vi "Main.vi"() -> ()   [LabVIEW 2024]
doc: "Use this template to build a simple state machine design pattern. Each state executes code and determines which state to transition to."
uses:
  controls/Valves--cluster.ctl
  controls/Controls--cluster.ctl
  controls/Sensors--cluster.ctl
  controls/SystemInfo--cluster.ctl
  <vilib>/gRPC/LabVIEW gRPC Library/Shared/grpcId.ctl
  controls/UI Queue Element.ctl
  controls/States.ctl
  controls/Stream Queue Element.ctl
  controls/Stream Loop States.ctl
  pumploop_client/RPC Messages/pumploop_GetSysInfRequest.ctl
  pumploop_client/RPC Messages/pumploop_GetValveRequest.ctl
  pumploop_client/RPC Messages/pumploop_GetControlRequest.ctl
  pumploop_client/RPC Messages/pumploop_Controls.ctl
  pumploop_client/RPC Messages/pumploop_Valves.ctl
  pumploop_client/RPC Messages/pumploop_GetSensorRequest.ctl
  pumploop_client/pumploop_client.lvlib
  <vilib>/gRPC/LabVIEW gRPC Library/grpc-lvsupport-release.lvlib
  pumploop_client/RPC Messages/pumploop_SystemInfo.ctl
panel:
  out "Read Attempts":i32
  out "Successes":bool[](array[boolean])
  in  "Apply Preset":bool
  in  "Address Presets":enum16{"Home WiFi", "RasPi WiFi"}(ring)
  out "Stream Status":string
  out "Stream Response Graph":waveform(dbl)[](graph)
  in  "Stream Enable":bool
  out "Node Info":T1
  out "Sensors":T2 {"Pump Speed" scale=0.0..10.0; "Ambient Pressure" scale=0.5..1.5; "DUT Outlet Pressure" scale=0.0..5.0; "DUT Inlet Pressure" scale=0.0..10.0; "Flow" scale=0.0..100.0; "Sump Level" scale=0.0..100.0; "Tank Level" scale=0.0..100.0; "DUT Temp" scale=0.0..150.0; "Pump Temp" scale=0.0..150.0; "Tank Temp" scale=0.0..100.0; "Ambient Temp" scale=0.0..50.0}
  in  "Get/Set":enum16{"Get", "Set"}(ring)
  in  "Subsystem":T3(ring)
  in  "Stream":enum16{"Disabled", "Enabled"}(ring)
  in  "Stop":bool
  in  "gRPC Disconnect":bool
  in  "Server Address":string="10.42.0.1:50051"
  in  "gRPC Connect":bool
  in  "Pump Control":T4
  in  "Control Valves":T5
  out "gRPC ID Out":u64
  out "Error":errorcluster
  # "Open"
  # "Closed"
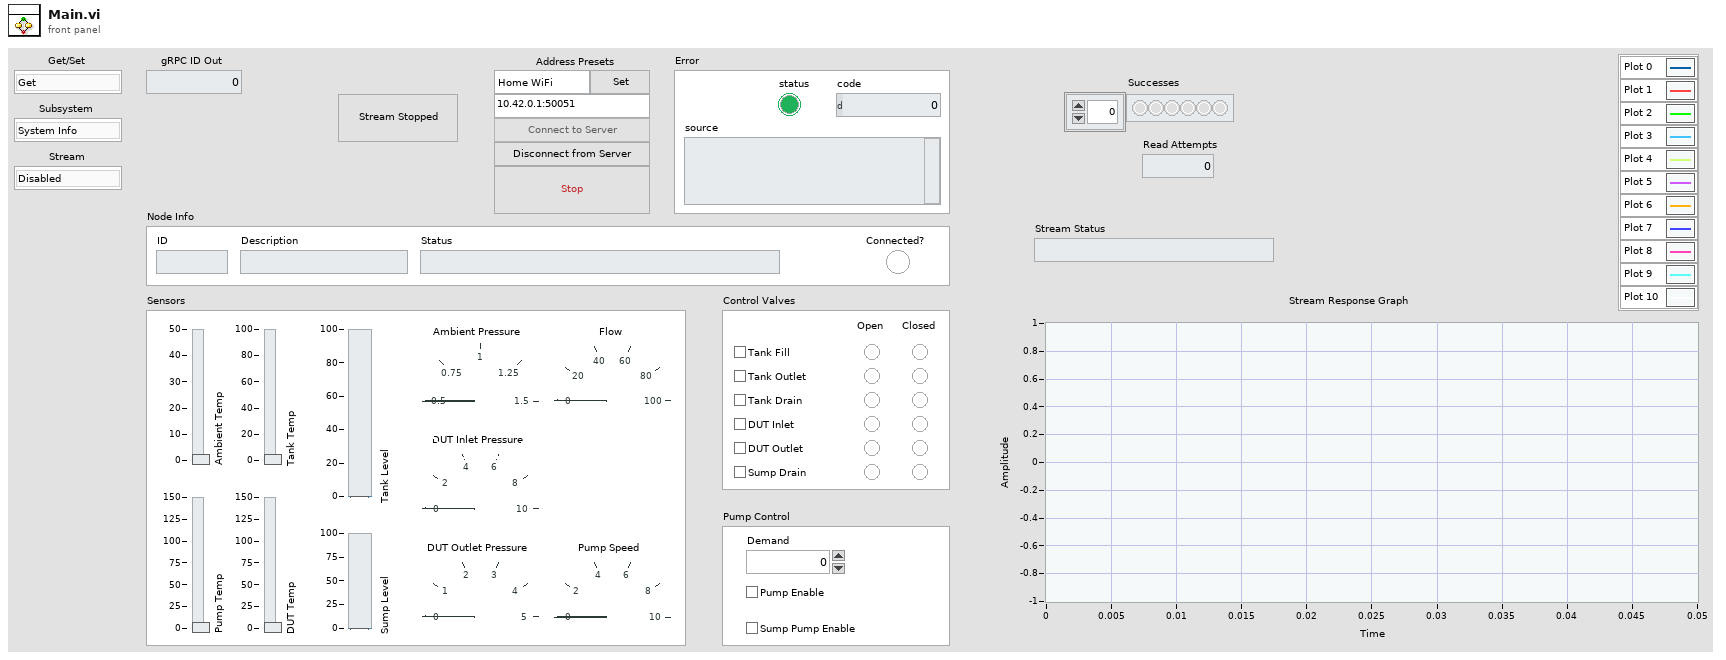
[diagram p1: front panel]
types:
  T1 = typedef "SystemInfo--cluster.ctl" = cluster{"Connected?":bool, "ID":string, "Description":string, "Status":string}
  T2 = typedef "Sensors--cluster.ctl" = cluster{"Tank Level":dbl, "Tank Temp":dbl, "Flow":dbl, "Pump Temp":dbl, "Pump Speed":dbl, "DUT Inlet Pressure":dbl, "DUT Outlet Pressure":dbl, "DUT Temp":dbl, "Sump Level":dbl, "Ambient Temp":dbl, "Ambient Pressure":dbl}
  T3 = enum16{"System Info", "Valves", "Sensors", "Control"}
  T4 = typedef "Controls--cluster.ctl" = cluster{"Pump Enable":bool, "Demand":dbl, "Sump Pump Enable":bool}
  T5 = typedef "Valves--cluster.ctl" = cluster{"Tank Fill":bool, "Tank Outlet":bool, "Tank Drain":bool, "DUT Inlet":bool, "DUT Outlet":bool, "Sump Drain":bool, "Tank Fill Open":bool, "Tank Fill Closed":bool, "Tank Outlet Open":bool, "Tank Outlet Closed":bool, "Tank Drain Open":bool, "Tank Drain Closed":bool, "DUT Inlet Open":bool, "DUT Inlet Closed":bool, "DUT Outlet Open":bool, "DUT Outlet Closed":bool, "Sump Drain Open":bool, "Sump Drain Closed":bool}
  T6 = typedef "grpc-lvsupport-release.lvlib/grpcId.ctl" = u64
  T7 = cluster{"Server Connected?":bool, "Streaming?":bool, "gRPC ID":T6, "Call Id":T6, "Stream Loop Status":string}
  T8 = typedef "Stream Loop States.ctl" = enum16{"Initialise", "gRPC_Connected", "gRPC_Disconnected", "gRPC_StartStream", "gRPC_Streaming", "gRPC_StopStream", "Update Settings", "Stop", "Quit"}
  T9 = typedef "Stream Queue Element.ctl" = cluster{"Enum":T8, variant}
  T10 = typedef "States.ctl" = enum16{"Initialise", "gRPC_Connect", "gRPC_Disconnect", "gRPC_Update-PumpCtrl", "gRPC_Update-ValveCtrl", "gRPC_ReadAll", "gRPC_Stream-Start", "gRPC_Stream-Stop", "Update Settings", "Stop", "Quit"}
  T11 = typedef "UI Queue Element.ctl" = cluster{T10, variant}
  T12 = cluster{"Node Info":T1, "Control Valves":T5, "Pump Control":T4, "Sensors":T2, "address":string, "Streaming":bool}
  T13 = typedef "pumploop_client.lvlib/pumploop_GetSysInfRequest.ctl" = cluster{"request":bool}
  T14 = typedef "pumploop_client.lvlib/pumploop_SystemInfo.ctl" = cluster{"nodeID":i32, "nodeDescription":string, "statusMsg":string}
  T15 = typedef "pumploop_client.lvlib/pumploop_GetValveRequest.ctl" = cluster{"request":bool}
  T16 = typedef "pumploop_client.lvlib/pumploop_Valves.ctl" = cluster{"tankFillIV":bool, "tankOutIV":bool, "tankDrainIV":bool, "dutInIV":bool, "dutOutIV":bool, "sumpDrainIV":bool}
  T17 = typedef "pumploop_client.lvlib/pumploop_GetSensorRequest.ctl" = cluster{"request":bool}
  T18 = typedef "pumploop_client.lvlib/pumploop_GetControlRequest.ctl" = cluster{"request":bool}
  T19 = typedef "pumploop_client.lvlib/pumploop_Controls.ctl" = cluster{"pumpEnable":bool, "pumpDemand":sgl, "sumppumpEnable":bool}
  T20 = typedef "pumploop_client.lvlib/pumploop_Sensors.ctl" = cluster{"tankLevel":sgl, "tankTemp":sgl, "dutFlow":sgl, "pumpTemp":sgl, "pumpSpeed":sgl, "dutPressIn":sgl, "dutPressOut":sgl, "dutTemp":sgl, "sumpLevel":sgl, "ambientTemp":sgl, "ambientPress":sgl}
  T21 = enum8{"Enabled", "Disabled", "Disabled and Grayed Out"}
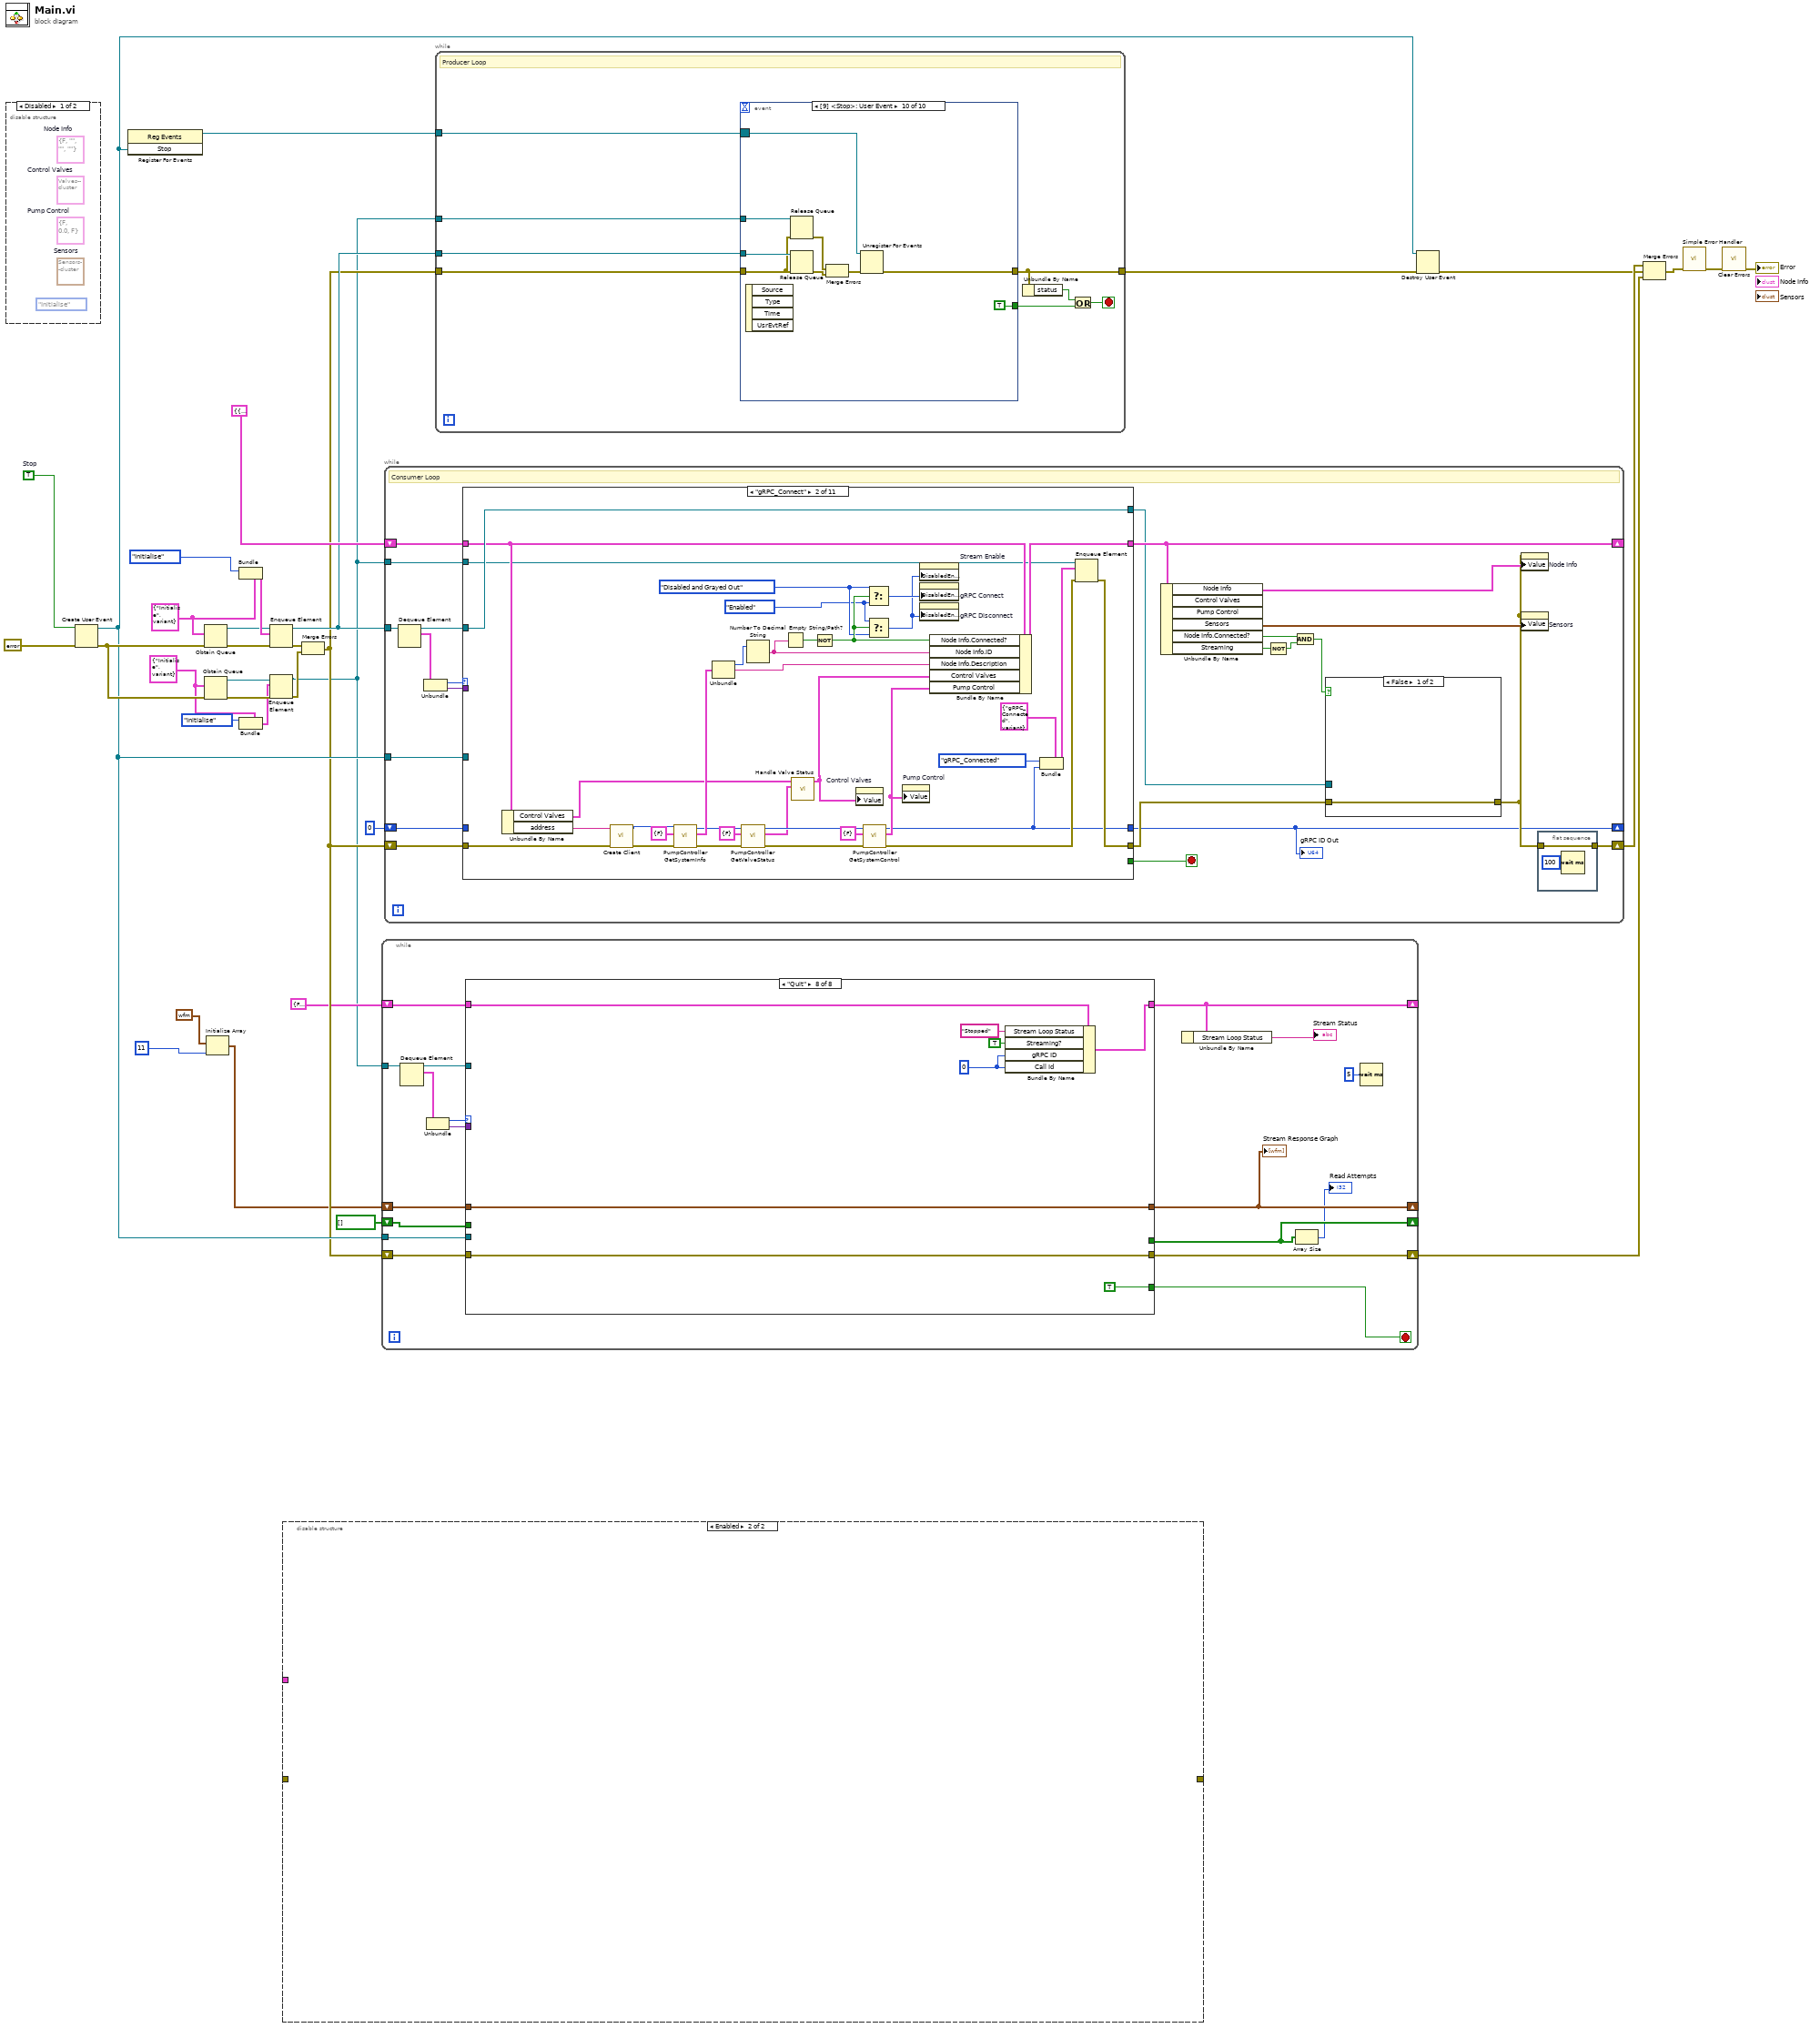
[diagram p0: block diagram]
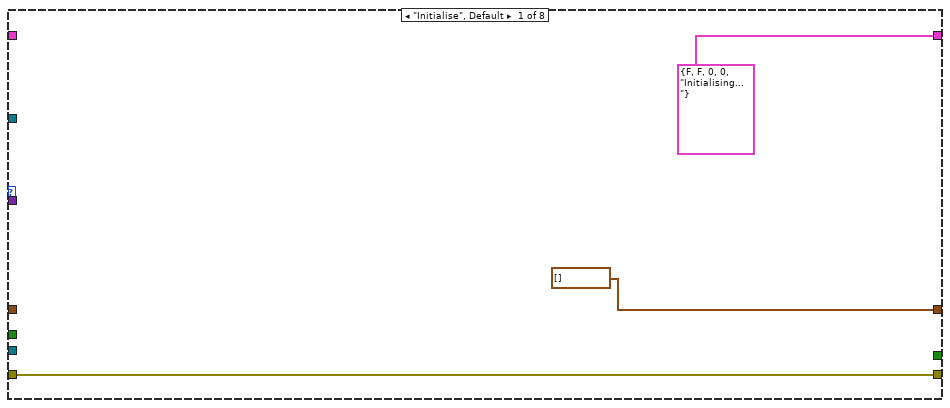
[diagram p2: hidden frame]
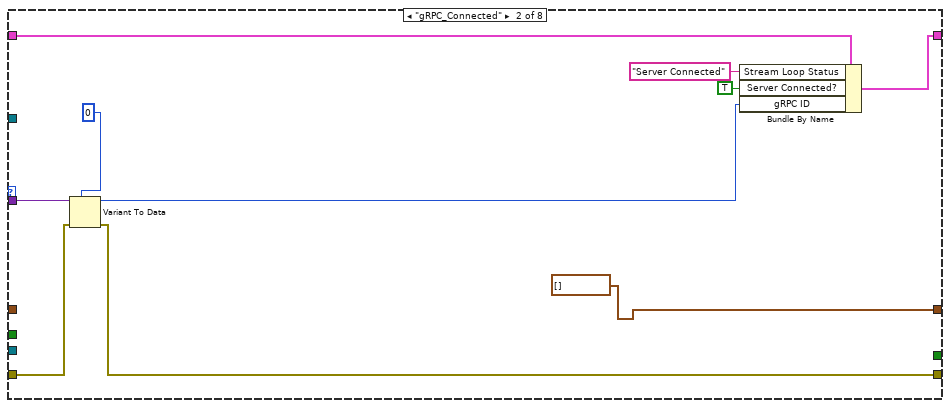
[diagram p3: hidden frame]
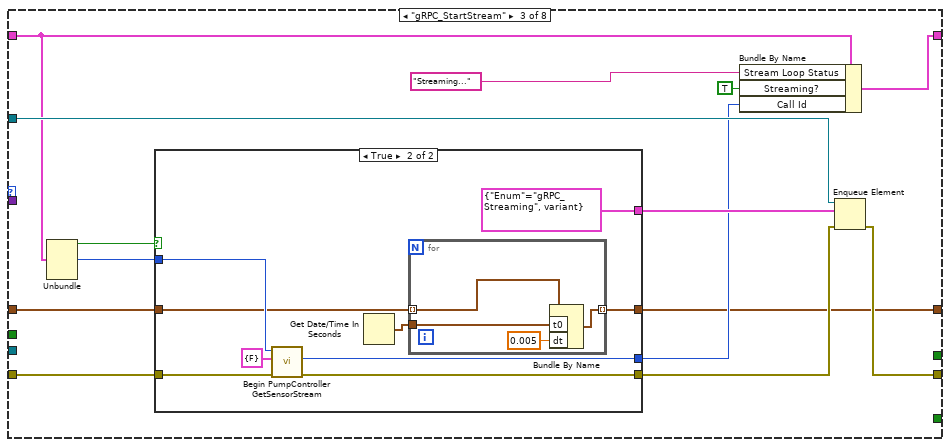
[diagram p4: hidden frame]
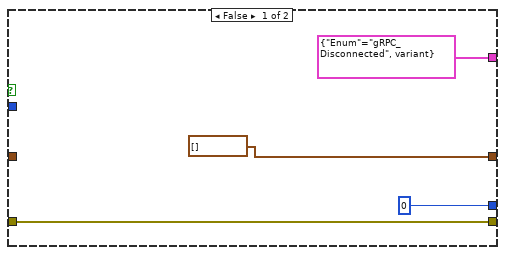
[diagram p5: hidden frame]
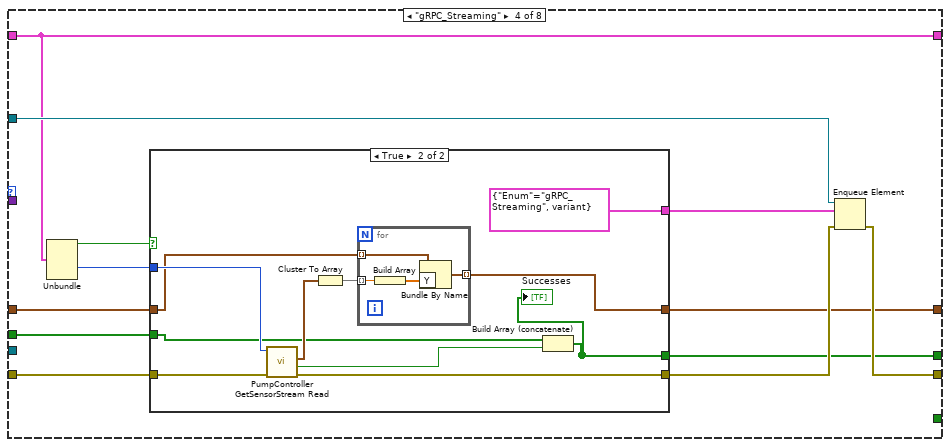
[diagram p6: hidden frame]
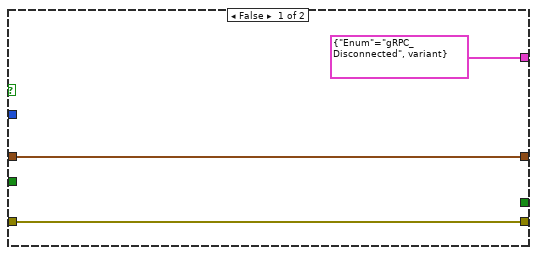
[diagram p7: hidden frame]
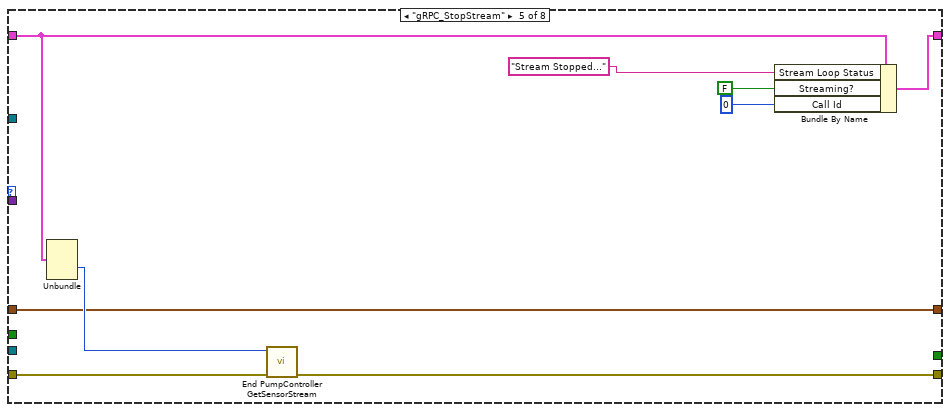
[diagram p8: hidden frame]
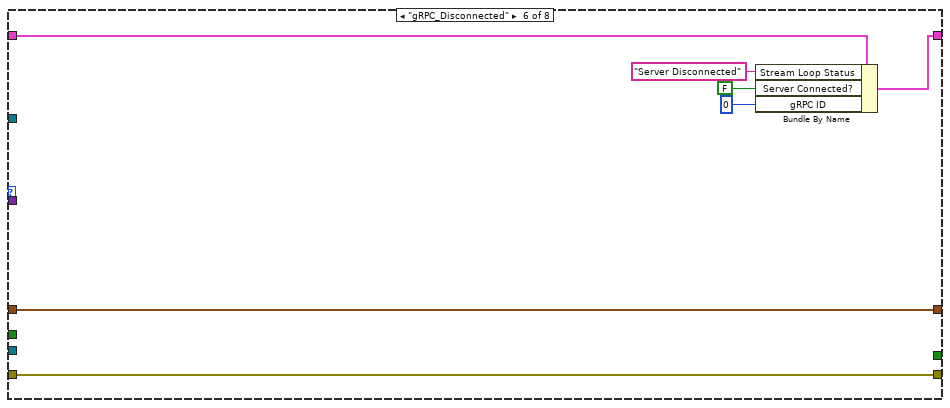
[diagram p9: hidden frame]
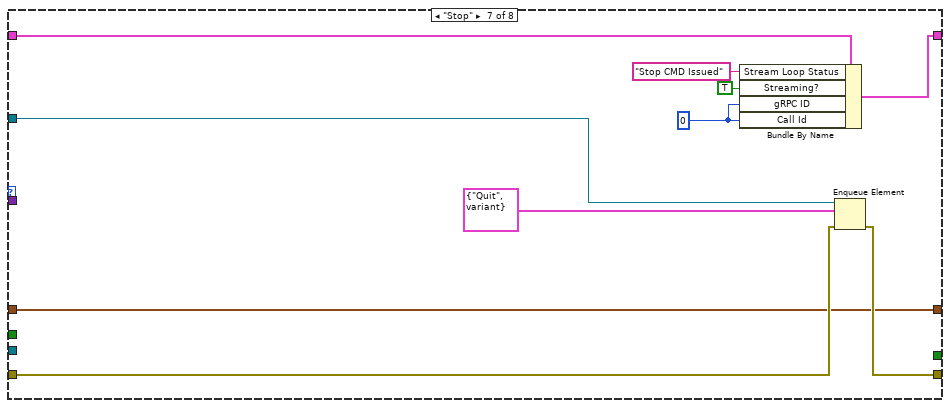
[diagram p10: hidden frame]
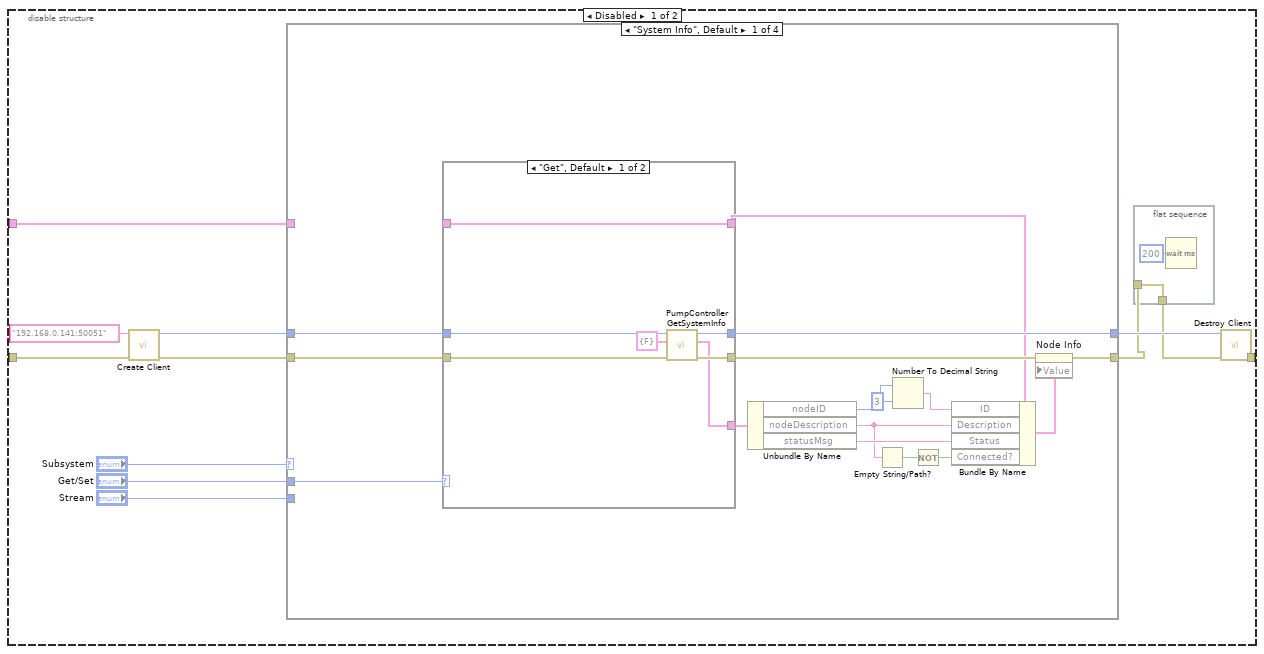
[diagram p12: hidden frame]
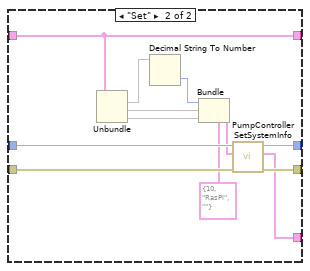
[diagram p13: hidden frame]
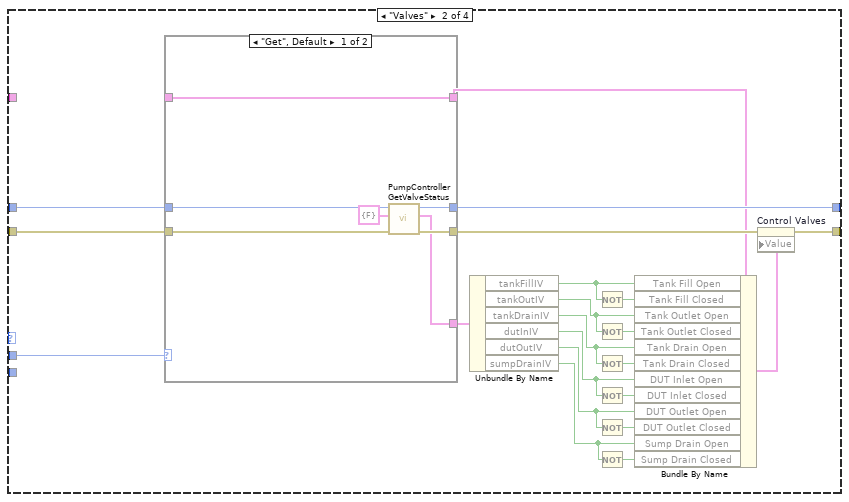
[diagram p14: hidden frame]
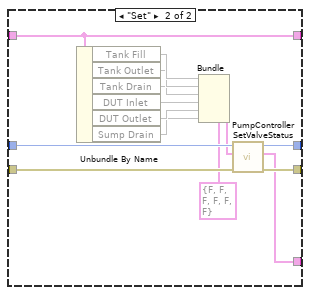
[diagram p15: hidden frame]
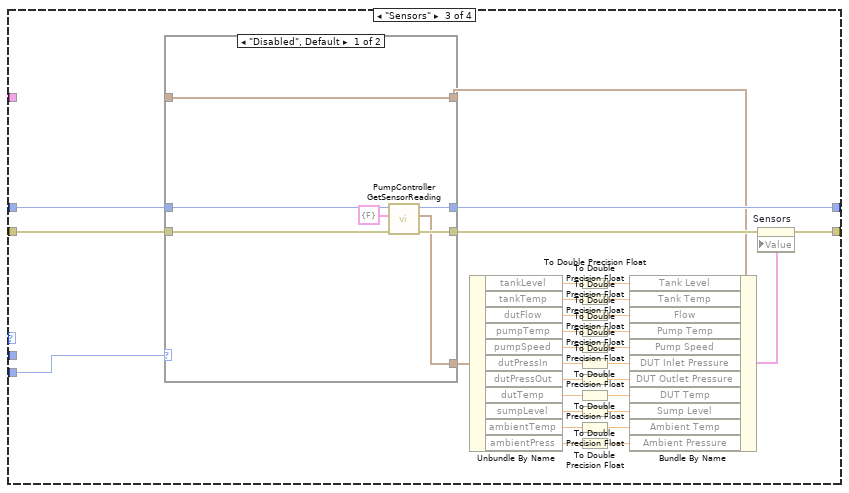
[diagram p16: hidden frame]
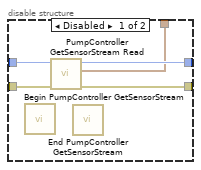
[diagram p18: hidden frame]
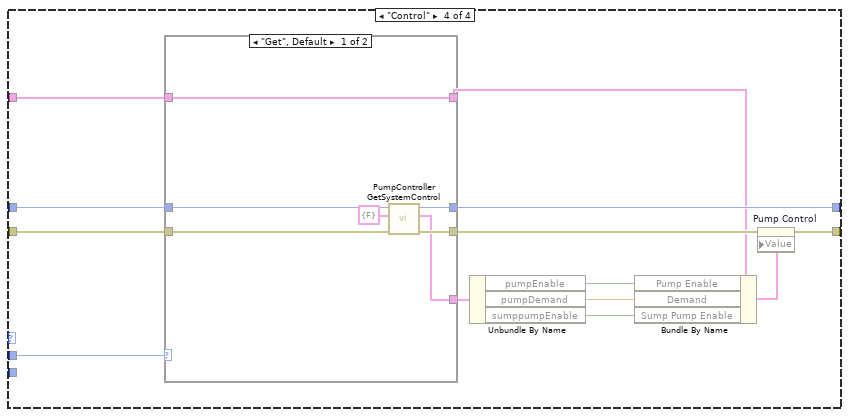
[diagram p19: hidden frame]
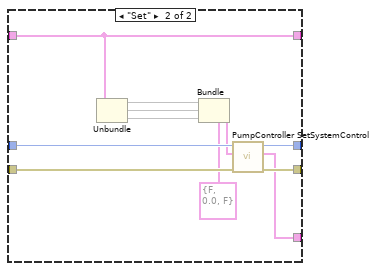
[diagram p20: hidden frame]
diagram:
  w14 = T9 {"Enum"=enum."Initialise", variant}
  w23 = TRUE  # Stop
  w11 = T11 {enum."Initialise", variant}
  n1 = disable-structure shown="Disabled" {
    frame Disabled {
      (unwired) States."Initialise"
      (unwired) T2 {"Tank Level"=0.0, "Tank Temp"=0.0, "Flow"=0.0, "Pump Temp"=0.0, "Pump Speed"=0.0, "DUT Inlet Pressure"=0.0, "DUT Outlet Pressure"=0.0, "DUT Temp"=0.0, "Sump Level"=0.0, "Ambient Temp"=0.0, "Ambient Pressure"=0.0}  # Sensors
      (unwired) T4 {"Pump Enable"=FALSE, "Demand"=0.0, "Sump Pump Enable"=FALSE}  # Pump Control
      (unwired) T5 {"Tank Fill"=FALSE, "Tank Outlet"=FALSE, "Tank Drain"=FALSE, "DUT Inlet"=FALSE, "DUT Outlet"=FALSE, "Sump Drain"=FALSE, "Tank Fill Open"=FALSE, "Tank Fill Closed"=FALSE, "Tank Outlet Open"=FALSE, "Tank Outlet Closed"=FALSE, "Tank Drain Open"=FALSE, "Tank Drain Closed"=FALSE, "DUT Inlet Open"=FALSE, "DUT Inlet Closed"=FALSE, "DUT Outlet Open"=FALSE, "DUT Outlet Closed"=FALSE, "Sump Drain Open"=FALSE, "Sump Drain Closed"=FALSE}  # Control Valves
      (unwired) T1 {"Connected?"=FALSE, "ID"="", "Description"="", "Status"=""}  # Node Info
    }
    frame Enabled {
    }
  }
  n2 = Create User Event(user event datatype=w23, error in=errorcluster {"status"=FALSE, "code"=0, "source"=""}) -> (user event=w16:refnum<user-event>, error out=w17:errorcluster)
  n3 = register-events(w16) -> (reference out=w21:refnum<event-registration>)  [unwired: 2 in, 1 out]
  n4 = Obtain Queue(element data type=w11, error in (no error)=w17) -> (queue out=w27:refnum<queue>, error out=w26:errorcluster)  [unwired: 3 in, 1 out]
  n5 = Obtain Queue(element data type=w14, error in (no error)=w17) -> (queue out=w15:refnum<queue>, error out=w18:errorcluster)  [unwired: 3 in, 1 out]
  n6 = Initialize Array(waveform(dbl) {"t0"=timestamp(0 s since 1904-01-01), "dt"=1.0, "Y"=[]} ("waveform"), 11 ("dimension size")) -> (w2:waveform(dbl)[])
  n7 = Bundle(cluster=w11, States."Initialise") -> (w29:T11)  [unwired: 1 in]
  n8 = Bundle(cluster=w14, "Enum"=Stream_Loop_States."Initialise") -> (w12:T9)  [unwired: 1 in]
  n9 = Enqueue Element(queue=w27, element=w29, error in (no error)=w26) -> (queue out=w25:refnum<queue>, error out=w10:errorcluster)  [unwired: 1 in, 1 out]
  n10 = Enqueue Element(queue=w15, element=w12, error in (no error)=w18) -> (queue out=w1:refnum<queue>, error out=w9:errorcluster)  [unwired: 1 in, 1 out]
  n11 = disable-structure shown="Enabled" {
    disable-tunnel: [w39 _] -> _
    disable-tunnel: _ -> [w36 _]
    disable-tunnel: _ -> [w35 _]
    frame Disabled {
      n12 = call "Create Client.vi"("error in"=w36, "address"="192.168.0.141:50051") -> ("error out"=w46:errorcluster, "gRPC ID Out"=w44:T6)  [unwired: 8 in]
      n13 = case shown="\"System Info\", Default" "Subsystem" {
        tunnel: w46 -> [w64 w104 w156 w187]
        tunnel: [w59 w100 w127 w179] -> w38
        tunnel: [w63 w103 w155 w186] -> w45
        tunnel: w44 -> [w62 w102 w154 w185]
        tunnel: "Get/Set" -> [w61 w101 _ w184]
        tunnel: "Stream" -> [_ _ w153 _]
        tunnel: w35 -> [_ _ _ w175]
        frame "System Info", Default {
          n14 = case shown="\"Get\", Default" w61 {
            tunnel: w64 -> [w71 w83]
            tunnel: [w69 w82] -> w60
            tunnel: [w68 w81] -> w63
            tunnel: w62 -> [w70 w80]
            tunnel: [w67 w79] -> w58
            tunnel: _ -> [w65 w77]
            tunnel: [w65 w77] -> w52
            frame "Get", Default {
              n15 = call "PumpController GetSystemInfo.vi"("error in"=w71, "Request Data"=T13 {"request"=FALSE}, "gRPC ID"=w70) -> ("error out"=w69:errorcluster, "Response Data"=w67:T14, "gRPC ID out"=w68:T6)  [unwired: 6 in]
            }
            frame "Set" {
              n16 = Unbundle(w77) -> ("ID"=w73, "Description"=w75, "Status"=w74)  [unwired: 1 out]
              n17 = Decimal String To Number(string=w73) -> (number=w72:i32)  [unwired: 2 in, 1 out]
              n18 = Bundle(cluster=T14 {"nodeID"=10, "nodeDescription"="RasPi", "statusMsg"=""} ("Node Info Request"), "nodeID"=w72, "nodeDescription"=w75, "statusMsg"=w74) -> (w76:T14)
              n19 = call "PumpController SetSystemInfo.vi"("error in"=w83, "Request Data"=w76, "gRPC ID"=w80) -> ("error out"=w82:errorcluster, "Response Data"=w79:T14, "gRPC ID out"=w81:T6)  [unwired: 6 in]
            }
          }
          n20 = Unbundle By Name(w58) -> ("nodeID"=w55:i32, "nodeDescription"=w51:string, "statusMsg"=w56:string)
          n21 = Empty String/Path?(string/path=w51) -> (empty?=w50:bool)
          n22 = Number To Decimal String(number=w55, width (-)=i16 3) -> (decimal integer string=w54:string)
          n23 = Not(x=w50) -> (.not. x?=w49:bool)
          n24 = Bundle By Name(cluster=w52, "ID"=w54, "Description"=w51, "Status"=w56, "Connected?"=w49) -> (w57:cluster{})
          n25 = property on="Node Info" class="Clust (strict)"(error in=w60, "Value"=w57) -> (error out=w59:errorcluster)  [unwired: 1 in, 1 out]
        }
        frame "Valves" {
          n26 = case shown="\"Get\", Default" w101 {
            tunnel: w104 -> [w110 w124]
            tunnel: [w109 w122] -> w99
            tunnel: [w108 w123] -> w103
            tunnel: w102 -> [w111 w125]
            tunnel: [w107 w121] -> w98
            tunnel: _ -> [w105 w112]
            tunnel: [w105 w112] -> w84
            frame "Get", Default {
              n27 = call "PumpController GetValveStatus.vi"("error in"=w110, "Request Data"=T15 {"request"=FALSE}, "gRPC ID"=w111) -> ("error out"=w109:errorcluster, "Response Data"=w107:T16, "gRPC ID out"=w108:T6)  [unwired: 6 in]
            }
            frame "Set" {
              n28 = Unbundle By Name(w112) -> ("Tank Fill"=w119, "Tank Outlet"=w118, "Tank Drain"=w117, "DUT Inlet"=w116, "DUT Outlet"=w115, "Sump Drain"=w114)
              n29 = Bundle(cluster=T16 {"tankFillIV"=FALSE, "tankOutIV"=FALSE, "tankDrainIV"=FALSE, "dutInIV"=FALSE, "dutOutIV"=FALSE, "sumpDrainIV"=FALSE} ("Valve Control Request"), "tankFillIV"=w119, "tankOutIV"=w118, "tankDrainIV"=w117, "dutInIV"=w116, "dutOutIV"=w115, "sumpDrainIV"=w114) -> (w113:T16)
              n30 = call "PumpController SetValveStatus.vi"("error in"=w124, "Request Data"=w113, "gRPC ID"=w125) -> ("error out"=w122:errorcluster, "Response Data"=w121:T16, "gRPC ID out"=w123:T6)  [unwired: 6 in]
            }
          }
          n31 = Unbundle By Name(w98) -> ("tankFillIV"=w89:bool, "tankOutIV"=w88:bool, "tankDrainIV"=w90:bool, "dutInIV"=w87:bool, "dutOutIV"=w86:bool, "sumpDrainIV"=w85:bool)
          n32 = Not(x=w89) -> (.not. x?=w96:bool)
          n33 = Not(x=w88) -> (.not. x?=w95:bool)
          n34 = Not(x=w90) -> (.not. x?=w94:bool)
          n35 = Not(x=w87) -> (.not. x?=w93:bool)
          n36 = Not(x=w86) -> (.not. x?=w92:bool)
          n37 = Not(x=w85) -> (.not. x?=w91:bool)
          n38 = Bundle By Name(cluster=w84, "Tank Fill Open"=w89, "Tank Fill Closed"=w96, "Tank Outlet Open"=w88, "Tank Outlet Closed"=w95, "Tank Drain Open"=w90, "Tank Drain Closed"=w94, "DUT Inlet Open"=w87, "DUT Inlet Closed"=w93, "DUT Outlet Open"=w86, "DUT Outlet Closed"=w92, "Sump Drain Open"=w85, "Sump Drain Closed"=w91) -> (w97:cluster{})
          n39 = property on="Control Valves" class="Clust (strict)"(error in=w99, "Value"=w97) -> (error out=w100:errorcluster)  [unwired: 1 in, 1 out]
        }
        frame "Sensors" {
          n40 = case shown="\"Disabled\", Default" w153 {
            tunnel: w156 -> [w160 w166]
            tunnel: [w162 w169] -> w128
            tunnel: [w163 w168] -> w155
            tunnel: w154 -> [w161 w167]
            tunnel: [w158 w165] -> w152
            tunnel: [w157 w164] -> w126
            tunnel: _ -> [w157 w164]
            frame "Disabled", Default {
              n41 = call "PumpController GetSensorReading.vi"("error in"=w160, "Request Data"=T17 {"request"=FALSE}, "gRPC ID"=w161) -> ("error out"=w162:errorcluster, "Response Data"=w158:T20, "gRPC ID out"=w163:T6)  [unwired: 6 in]
            }
            frame "Enabled" {
              n42 = disable-structure shown="Enabled" {
                disable-tunnel: [w174 _] -> w169
                disable-tunnel: [w173 _] -> w168
                disable-tunnel: w167 -> [w172 _]
                disable-tunnel: w166 -> [w171 _]
                disable-tunnel: [w170 _] -> w165
                frame Disabled {
                  n43 = call "Begin PumpController GetSensorStream.vi"() -> ()  [unwired: 9 in, 3 out]
                  n44 = call "PumpController GetSensorStream Read.vi"("error in"=w171, "Call ID in"=w172) -> ("error out"=w174:errorcluster, "Response Data"=w170:T20, "Call ID"=w173:T6)  [unwired: 6 in, 1 out]
                  n45 = call "End PumpController GetSensorStream.vi"() -> ()  [unwired: 10 in, 2 out]
                }
                frame Enabled {
                }
              }
            }
          }
          n46 = Unbundle By Name(w152) -> ("tankLevel"=w151:sgl, "tankTemp"=w150:sgl, "dutFlow"=w149:sgl, "pumpTemp"=w147:sgl, "pumpSpeed"=w146:sgl, "dutPressIn"=w148:sgl, "dutPressOut"=w145:sgl, "dutTemp"=w144:sgl, "sumpLevel"=w143:sgl, "ambientTemp"=w142:sgl, "ambientPress"=w141:sgl)
          n47 = To Double Precision Float(number=w151) -> (double precision float=w140:dbl)
          n48 = To Double Precision Float(number=w150) -> (double precision float=w139:dbl)
          n49 = To Double Precision Float(number=w149) -> (double precision float=w138:dbl)
          n50 = To Double Precision Float(number=w147) -> (double precision float=w137:dbl)
          n51 = To Double Precision Float(number=w146) -> (double precision float=w136:dbl)
          n52 = To Double Precision Float(number=w148) -> (double precision float=w135:dbl)
          n53 = To Double Precision Float(number=w145) -> (double precision float=w134:dbl)
          n54 = To Double Precision Float(number=w144) -> (double precision float=w133:dbl)
          n55 = To Double Precision Float(number=w143) -> (double precision float=w132:dbl)
          n56 = To Double Precision Float(number=w142) -> (double precision float=w131:dbl)
          n57 = To Double Precision Float(number=w141) -> (double precision float=w130:dbl)
          n58 = Bundle By Name(cluster=w126, "Tank Level"=w140, "Tank Temp"=w139, "Flow"=w138, "Pump Temp"=w137, "Pump Speed"=w136, "DUT Inlet Pressure"=w135, "DUT Outlet Pressure"=w134, "DUT Temp"=w133, "Sump Level"=w132, "Ambient Temp"=w131, "Ambient Pressure"=w130) -> (w129:cluster{})
          n59 = property on="Sensors" class="Clust (strict)"(error in=w128, "Value"=w129) -> (error out=w127:errorcluster)  [unwired: 1 in, 1 out]
        }
        frame "Control" {
          n60 = case shown="\"Get\", Default" w184 {
            tunnel: w187 -> [w193 w204]
            tunnel: [w191 w202] -> w178
            tunnel: [w192 w203] -> w186
            tunnel: w185 -> [w194 w205]
            tunnel: [w190 w201] -> w183
            tunnel: w175 -> [w188 w196]
            tunnel: [w188 w196] -> w176
            frame "Get", Default {
              n61 = call "PumpController GetSystemControl.vi"("error in"=w193, "Request Data"=T18 {"request"=FALSE}, "gRPC ID"=w194) -> ("error out"=w191:errorcluster, "Response Data"=w190:T19, "gRPC ID out"=w192:T6)  [unwired: 6 in]
            }
            frame "Set" {
              n62 = Unbundle(w196) -> ("Pump Enable"=w199, "Demand"=w200, "Sump Pump Enable"=w195)
              n63 = Bundle(cluster=T19 {"pumpEnable"=FALSE, "pumpDemand"=0.0, "sumppumpEnable"=FALSE} ("System Control Request"), "pumpEnable"=w199, "pumpDemand"=w200, "sumppumpEnable"=w195) -> (w198:T19)
              n64 = call "PumpController SetSystemControl.vi"("error in"=w204, "Request Data"=w198, "gRPC ID"=w205) -> ("error out"=w202:errorcluster, "Response Data"=w201:T19, "gRPC ID out"=w203:T6)  [unwired: 6 in]
            }
          }
          n65 = Unbundle By Name(w183) -> ("pumpEnable"=w182:bool, "pumpDemand"=w181:sgl, "sumppumpEnable"=w180:bool)
          n66 = Bundle By Name(cluster=w176, "Pump Enable"=w182, "Demand"=w181, "Sump Pump Enable"=w180) -> (w177:cluster{})
          n67 = property on="Pump Control" class="Clust (strict)"(error in=w178, "Value"=w177) -> (error out=w179:errorcluster)  [unwired: 1 in, 1 out]
        }
      }
      n68 = flat-sequence {
        tunnel: w38 -> [w48]
        tunnel: [w48] -> w37
        frame #0 {
          n69 = Wait (ms)(milliseconds to wait=u32 200) -> ()  [unwired: 1 out]
        }
      }
      n70 = call "Destroy Client.vi"("error in"=w37, "gRPC ID"=w45) -> ("error out"=w39:errorcluster)  [unwired: 9 in]
    }
    frame Enabled {
    }
  }
  n71 = Merge Errors(w10, w9) -> (w8:errorcluster)
  n72 = while {
    tunnel: w16 -> [w214]
    tunnel: w1 -> [w222]
    shift-right: [w220] -> w6
    shift-left: w8 -> [w219]
    shift-right: [w212] -> _
    shift-left: T7 {"Server Connected?"=FALSE, "Streaming?"=FALSE, "gRPC ID"=0, "Call Id"=0, "Stream Loop Status"=""} -> [w218]
    shift-right: [w208] -> _
    shift-left: w2 -> [w215]
    shift-right: [w207] -> _
    shift-left: bool[] [] -> [w209]
    stop <- w213 stop-if-true
    n73 = Dequeue Element(queue=w222) -> (queue out=w216:refnum<queue>, element=w223:T9)  [unwired: 2 in, 2 out]
    n74 = Unbundle(w223) -> ("Enum"=w221:T8, w217:variant)
    n75 = case shown="\"Quit\"" w221 {
      tunnel: [w226 w234 w248 w279 w300 w310 w321 w324] -> w220
      tunnel: w219 -> [w226 w235 w245 w276 w302 w310 w318 w324]
      tunnel: [T7 {"Server Connected?"=FALSE, "Streaming?"=FALSE, "gRPC ID"=0, "Call Id"=0, "Stream Loop Status"="Initialising..."} w232 w250 w272 w306 w312 w323 w331] -> w212
      tunnel: w218 -> [_ w233 w243 w272 w304 w313 w317 w329]
      tunnel: w217 -> [_ w236 _ _ _ _ _ _]
      tunnel: w216 -> [_ _ w247 w278 _ _ w320 _]
      tunnel: [waveform(dbl)[] [] ("initialized array") waveform(dbl)[] [] ("initialized array") w237 w270 w299 w308 w315 w327] -> w208
      tunnel: w215 -> [_ _ w238 w271 w299 w308 w315 w327]
      tunnel: w214 -> [_ _ _ _ _ _ _ _]
      tunnel: [_ _ _ _ _ _ _ TRUE] -> w213
      tunnel: [_ _ _ w269 _ _ _ _] -> w207
      tunnel: w209 -> [_ _ _ w268 _ _ _ _]
      frame "Initialise", Default {
      }
      frame "gRPC_Connected" {
        n76 = Variant To Data(error in=w235, type=T6 0 ("gRPC ID Out"), Variant=w236) -> (data=w231:T6, error out=w234:errorcluster)
        n77 = Bundle By Name(cluster=w233, "Stream Loop Status"="Server Connected", "Server Connected?"=TRUE, "gRPC ID"=w231) -> (w232:T7)
      }
      frame "gRPC_StartStream" {
        n78 = Unbundle(w243) -> ("Server Connected?"=w242:bool, "gRPC ID"=w241:T6)  [unwired: 3 out]
        n79 = case shown="True" w242 {
          tunnel: [T9 {"Enum"=enum."gRPC_Disconnected", variant} ("element") T9 {"Enum"=enum."gRPC_Streaming", variant} ("element")] -> w246
          tunnel: w245 -> [w253 w262]
          tunnel: [w253 w261] -> w244
          tunnel: w241 -> [_ w259]
          tunnel: [T6 0 ("Call Id Out") w258] -> w240
          tunnel: w238 -> [_ w257]
          tunnel: [waveform(dbl)[] [] ("initialized array") w256] -> w237
          frame False {
          }
          frame True {
            n80 = call "Begin PumpController GetSensorStream.vi"("error in"=w262, "Request Data"=T17 {"request"=FALSE}, "gRPC ID"=w259) -> ("error out"=w261:errorcluster, "Call Id Out"=w258:T6)  [unwired: 6 in, 1 out]
            n81 = Get Date/Time In Seconds() -> (seconds since 1Jan1904=w255:timestamp)
            n82 = for {
              tunnel: w257 -> [w267] mode=indexing
              tunnel: [w265] -> w256 mode=indexing
              tunnel: w255 -> [w264]
              n83 = Bundle By Name(cluster=w267, "t0"=w264, "dt"=0.005) -> (w265:waveform(dbl))
            }
          }
        }
        n84 = Bundle By Name(cluster=w243, "Stream Loop Status"="Streaming..." ("Node Info.Status"), "Streaming?"=TRUE ("Server Connected?"), "Call Id"=w240) -> (w250:T7)
        n85 = Enqueue Element(queue=w247, element=w246, error in (no error)=w244) -> (error out=w248:errorcluster)  [unwired: 1 in, 2 out]
      }
      frame "gRPC_Streaming" {
        n86 = Unbundle(w272) -> ("Server Connected?"=w274:bool, "Call Id"=w273:T6)  [unwired: 3 out]
        n87 = case shown="True" w274 {
          tunnel: [T9 {"Enum"=enum."gRPC_Disconnected", variant} ("element") T9 {"Enum"=enum."gRPC_Streaming", variant} ("element")] -> w277
          tunnel: w276 -> [w282 w291]
          tunnel: [w282 w292] -> w275
          tunnel: w273 -> [_ w290]
          tunnel: [w280 w288] -> w270
          tunnel: w271 -> [w280 w289]
          tunnel: [_ w283] -> w269
          tunnel: w268 -> [_ w284]
          frame False {
          }
          frame True {
            n88 = call "PumpController GetSensorStream Read.vi"("error in"=w291, "Call ID in"=w290) -> ("error out"=w292:errorcluster, "Success"=w285:bool, "Response Data"=w287:T20)  [unwired: 6 in, 1 out]
            n89 = Cluster To Array(cluster=w287) -> (array=w286:sgl[])
            n90 = for {
              tunnel: w289 -> [w297] mode=indexing
              tunnel: [w296] -> w288 mode=indexing
              tunnel: w286 -> [w295] mode=indexing
              n91 = Build Array(w295) -> (w294:sgl[])
              n92 = Bundle By Name(cluster=w297, "Y"=w294) -> (w296:waveform(dbl))
            }
            n93 = Build Array (concatenate)(w284, w285) -> (w283:bool[])
            "Successes" <- w283
          }
        }
        n94 = Enqueue Element(queue=w278, element=w277, error in (no error)=w275) -> (error out=w279:errorcluster)  [unwired: 1 in, 2 out]
      }
      frame "gRPC_StopStream" {
        n95 = Unbundle(w304) -> ("Call Id"=w301:T6)  [unwired: 4 out]
        n96 = call "End PumpController GetSensorStream.vi"("error in"=w302, "Call ID in"=w301) -> ("error out"=w300:errorcluster)  [unwired: 8 in, 1 out]
        n97 = Bundle By Name(cluster=w304, "Stream Loop Status"="Stream Stopped..." ("Node Info.Status"), "Streaming?"=FALSE ("Server Connected?"), "Call Id"=T6 0 ("Call Id Out")) -> (w306:T7)
      }
      frame "gRPC_Disconnected" {
        n98 = Bundle By Name(cluster=w313, "Stream Loop Status"="Server Disconnected", "Server Connected?"=FALSE, "gRPC ID"=T6 0) -> (w312:T7)
      }
      frame "Stop" {
        w316 = T6 0 ("Call Id Out")
        n99 = Bundle By Name(cluster=w317, "Stream Loop Status"="Stop CMD Issued", "Streaming?"=TRUE ("Server Connected?"), "gRPC ID"=w316, "Call Id"=w316) -> (w323:T7)
        n100 = Enqueue Element(queue=w320, element=T9 {"Enum"=enum."Quit", variant}, error in (no error)=w318) -> (error out=w321:errorcluster)  [unwired: 1 in, 2 out]
      }
      frame "Quit" {
        w328 = T6 0 ("Call Id Out")
        n101 = Bundle By Name(cluster=w329, "Stream Loop Status"="Stopped", "Streaming?"=TRUE ("Server Connected?"), "gRPC ID"=w328, "Call Id"=w328) -> (w331:T7)
      }
    }
    "Stream Response Graph" <- w208
    n102 = Unbundle By Name(w212) -> ("Stream Loop Status"=→"Stream Status":string)
    n103 = Array Size(array=w207) -> (size(s)=→"Read Attempts":i32)
    n104 = Wait (ms)(milliseconds to wait=u32 5) -> ()  [unwired: 1 out]
  }
  n105 = while {
    shift-right: [w340] -> w32
    shift-left: w8 -> [w354]
    shift-right: [w338] -> _
    shift-left: T6 0 ("gRPC ID Out") -> [w353]
    tunnel: w25 -> [w352]
    shift-right: [w346] -> _
    shift-left: T12 {"Node Info"={"Connected?"=FALSE, "ID"="", "Description"="", "Status"=""}, "Control Valves"={"Tank Fill"=FALSE, "Tank Outlet"=FALSE, "Tank Drain"=FALSE, "DUT Inlet"=FALSE, "DUT Outlet"=FALSE, "Sump Drain"=FALSE, "Tank Fill Open"=FALSE, "Tank Fill Closed"=FALSE, "Tank Outlet Open"=FALSE, "Tank Outlet Closed"=FALSE, "Tank Drain Open"=FALSE, "Tank Drain Closed"=FALSE, "DUT Inlet Open"=FALSE, "DUT Inlet Closed"=FALSE, "DUT Outlet Open"=FALSE, "DUT Outlet Closed"=FALSE, "Sump Drain Open"=FALSE, "Sump Drain Closed"=FALSE}, "Pump Control"={"Pump Enable"=FALSE, "Demand"=0.0, "Sump Pump Enable"=FALSE}, "Sensors"={"Tank Level"=0.0, "Tank Temp"=0.0, "Flow"=0.0, "Pump Temp"=0.0, "Pump Speed"=0.0, "DUT Inlet Pressure"=0.0, "DUT Outlet Pressure"=0.0, "DUT Temp"=0.0, "Sump Level"=0.0, "Ambient Temp"=0.0, "Ambient Pressure"=0.0}, "address"="192.168.0.141:50051", "Streaming"=FALSE} -> [w347]
    tunnel: w16 -> [w337]
    tunnel: w1 -> [w336]
    stop <- w343 stop-if-true
    # "Consumer Loop"
    n106 = Dequeue Element(queue=w352) -> (queue out=w349:refnum<queue>, element=w351:T11)  [unwired: 2 in, 2 out]
    n107 = Unbundle(w351) -> (w350:T10, w348:variant)
    n108 = case shown="\"gRPC_Connect\"" w350 {
      tunnel: w354 -> [w371 w409 w423 w430 w437 w458 w468 w498 w534 w564 w573]
      tunnel: [w371 w382 w412 w429 w440 w457 w471 w495 w533 w563 w572] -> w339
      tunnel: [w374 w378 T6 0 ("gRPC ID Out") w436 w439 w463 w470 w494 w532 w557 w566] -> w338
      tunnel: w353 -> [w374 _ w422 w436 w439 w463 w472 w496 w531 w557 w566]
      tunnel: w349 -> [w373 w408 w420 w435 w443 w460 w466 w493 w529 w565 w574]
      tunnel: w348 -> [_ _ _ w432 _ _ w469 w499 _ _ _]
      tunnel: w347 -> [_ w402 w415 w434 w438 w462 w465 w491 w528 w560 w569]
      tunnel: [w367 w401 w419 w433 w438 w462 w467 w497 w530 w559 w568] -> w346
      tunnel: [_ _ _ _ _ TRUE _ _ _ _ _] -> w343
      tunnel: [w373 w408 w420 w435 w443 w460 w466 w493 w529 w565 w574] -> w342
      tunnel: w337 -> [_ _ _ _ _ w459 _ _ _ _ _]
      tunnel: w336 -> [_ w381 w414 _ _ _ _ _ _ w562 w571]
      frame "Initialise", Default {
        w367 = T12 {"Node Info"={"Connected?"=FALSE, "ID"="", "Description"="", "Status"=""}, "Control Valves"={"Tank Fill"=FALSE, "Tank Outlet"=FALSE, "Tank Drain"=FALSE, "DUT Inlet"=FALSE, "DUT Outlet"=FALSE, "Sump Drain"=FALSE, "Tank Fill Open"=FALSE, "Tank Fill Closed"=FALSE, "Tank Outlet Open"=FALSE, "Tank Outlet Closed"=FALSE, "Tank Drain Open"=FALSE, "Tank Drain Closed"=FALSE, "DUT Inlet Open"=FALSE, "DUT Inlet Closed"=FALSE, "DUT Outlet Open"=FALSE, "DUT Outlet Closed"=FALSE, "Sump Drain Open"=FALSE, "Sump Drain Closed"=FALSE}, "Pump Control"={"Pump Enable"=FALSE, "Demand"=0.0, "Sump Pump Enable"=FALSE}, "Sensors"={"Tank Level"=0.0, "Tank Temp"=0.0, "Flow"=0.0, "Pump Temp"=0.0, "Pump Speed"=0.0, "DUT Inlet Pressure"=0.0, "DUT Outlet Pressure"=0.0, "DUT Temp"=0.0, "Sump Level"=0.0, "Ambient Temp"=0.0, "Ambient Pressure"=0.0}, "address"="10.42.0.1:50051", "Streaming"=FALSE}
        w366 = T21."Disabled and Grayed Out" ("Disabled")
        n109 = Unbundle By Name(w367) -> ("Node Info"=w369:T1, "Control Valves"=w368:T5, "Pump Control"=w370:T4, "Sensors"=w365:T2, "address"=w364:string)
        n110 = property on="Stream Enable" class="Bool (strict)"("DisabledEnum"=w366) -> ()  [unwired: 2 in, 2 out]
        n111 = property on="gRPC Connect" class="Bool"(error in=w371, "DisabledEnum"=T21."Enabled" ("Disabled")) -> ()  [unwired: 1 in, 2 out]
        n112 = property on="gRPC Disconnect" class="Bool"(error in=w371, "DisabledEnum"=w366) -> ()  [unwired: 1 in, 2 out]
        n113 = property on="Node Info" class="Clust (strict)"("Value"=w369) -> ()  [unwired: 2 in, 2 out]
        n114 = property on="Control Valves" class="Clust (strict)"("Value"=w368) -> ()  [unwired: 2 in, 2 out]
        n115 = property on="Pump Control" class="Clust (strict)"("Value"=w370) -> ()  [unwired: 2 in, 2 out]
        n116 = property on="Sensors" class="Clust (strict)"("Value"=w365) -> ()  [unwired: 2 in, 2 out]
        n117 = property on="Server Address" class="Str"("Value"=w364) -> ()  [unwired: 2 in, 2 out]
      }
      frame "gRPC_Connect" {
        w394 = T21."Enabled" ("Disabled")
        w395 = T21."Disabled and Grayed Out" ("Disabled")
        n118 = Unbundle By Name(w402) -> ("Control Valves"=w385:T5, "address"=w407:string)
        n119 = call "Create Client.vi"("error in"=w409, "address"=w407) -> ("error out"=w399:errorcluster, "gRPC ID Out"=w398:T6)  [unwired: 8 in]
        n120 = call "PumpController GetSystemInfo.vi"("error in"=w399, "Request Data"=T13 {"request"=FALSE}, "gRPC ID"=w398) -> ("error out"=w391:errorcluster, "Response Data"=w403:T14, "gRPC ID out"=w390:T6)  [unwired: 6 in]
        n121 = Unbundle(w403) -> ("nodeID"=w406:i32, "nodeDescription"=w405:string)  [unwired: 1 out]
        n122 = call "PumpController GetValveStatus.vi"("error in"=w391, "Request Data"=T15 {"request"=FALSE}, "gRPC ID"=w390) -> ("error out"=w392:errorcluster, "Response Data"=w386:T16, "gRPC ID out"=w389:T6)  [unwired: 6 in]
        n123 = Number To Decimal String(number=w406) -> (decimal integer string=w404:string)  [unwired: 1 in]
        n124 = Empty String/Path?(string/path=w404) -> (empty?=w397:bool)
        n125 = call "Handle Valve Status.vi"("Response Data"=w386, "Control Valves in"=w385) -> ("Control Valves out"=w375:T5)  [unwired: 9 in]
        n126 = Not(x=w397) -> (.not. x?=w396:bool)
        n127 = property on="Control Valves" class="Clust (strict)"("Value"=w375) -> ()  [unwired: 2 in, 2 out]
        n128 = call "PumpController GetSystemControl.vi"("error in"=w392, "Request Data"=T18 {"request"=FALSE}, "gRPC ID"=w389) -> ("error out"=w383:errorcluster, "Response Data"=w384:T19, "gRPC ID out"=w378:T6)  [unwired: 6 in]
        n129 = Select(t=w395, s=w396, f=w394) -> (s? t:f=w393:T21)
        n130 = Select(t=w394, s=w396, f=w395) -> (s? t:f=w376:T21)
        n131 = property on="Pump Control" class="Clust (strict)"("Value"=w384) -> ()  [unwired: 2 in, 2 out]
        n132 = property on="Stream Enable" class="Bool (strict)"("DisabledEnum"=w376) -> ()  [unwired: 2 in, 2 out]
        n133 = property on="gRPC Connect" class="Bool"("DisabledEnum"=w393) -> ()  [unwired: 2 in, 2 out]
        n134 = property on="gRPC Disconnect" class="Bool"("DisabledEnum"=w376) -> ()  [unwired: 2 in, 2 out]
        n135 = Bundle By Name(cluster=w402, "Node Info.Connected?"=w396, "Node Info.ID"=w404, "Node Info.Description"=w405, "Control Valves"=w375, "Pump Control"=w384) -> (w401:T12)
        n136 = Bundle(cluster=T9 {"Enum"=enum."gRPC_Connected", variant} ("element"), "Enum"=Stream_Loop_States."gRPC_Connected", w378) -> (w377:T9)
        n137 = Enqueue Element(queue=w381, element=w377, error in (no error)=w383) -> (error out=w382:errorcluster)  [unwired: 1 in, 2 out]
      }
      frame "gRPC_Disconnect" {
        w410 = T21."Disabled and Grayed Out" ("Disabled")
        n138 = Unbundle By Name(w415) -> ("Node Info.Connected?"=w416:bool)
        n139 = case shown="True" w416 {
          tunnel: w423 -> [w424 w427]
          tunnel: w422 -> [_ w426]
          tunnel: [w424 w425] -> w413
          frame False {
          }
          frame True {
            n140 = call "Destroy Client.vi"("error in"=w427, "gRPC ID"=w426) -> ("error out"=w425:errorcluster)  [unwired: 9 in]
          }
        }
        n141 = Bundle By Name(cluster=w415, "Node Info.Connected?"=FALSE) -> (w419:T12)
        n142 = property on="Stream Enable" class="Bool (strict)"("DisabledEnum"=w410) -> ()  [unwired: 2 in, 2 out]
        n143 = property on="gRPC Connect" class="Bool"(error in=w413, "DisabledEnum"=T21."Enabled" ("Disabled")) -> ()  [unwired: 1 in, 2 out]
        n144 = property on="gRPC Disconnect" class="Bool"(error in=w413, "DisabledEnum"=w410) -> ()  [unwired: 1 in, 2 out]
        n145 = Enqueue Element(queue=w414, element=T9 {"Enum"=enum."gRPC_Disconnected", variant}, error in (no error)=w413) -> (error out=w412:errorcluster)  [unwired: 1 in, 2 out]
      }
      frame "Update Settings" {
        n146 = Variant To Data(error in=w430, type="", Variant=w432) -> (data=w428:string, error out=w429:errorcluster)
        n147 = Bundle By Name(cluster=w434, "address"=w428) -> (w433:T12)
        n148 = property on="Server Address" class="Str"(error in=w429, "Value"=w428) -> ()  [unwired: 1 in, 2 out]
      }
      frame "Stop" {
        w441 = T11 {enum."Initialise", variant}
        n149 = Bundle(cluster=w441, States."gRPC_Disconnect") -> (w447:T11)  [unwired: 1 in]
        n150 = disable-structure shown="Enabled" {
          disable-tunnel: w447 -> [w453 _]
          disable-tunnel: [w452 w454] -> w445
          disable-tunnel: [w451 w455] -> w444
          disable-tunnel: w443 -> [w450 w455]
          disable-tunnel: w437 -> [w449 w454]
          frame Disabled {
            n151 = Enqueue Element(queue=w450, element=w453, error in (no error)=w449) -> (queue out=w451:refnum<queue>, error out=w452:errorcluster)  [unwired: 1 in, 1 out]
          }
          frame Enabled {
          }
        }
        n152 = Bundle(cluster=w441, States."Quit") -> (w442:T11)  [unwired: 1 in]
        n153 = Enqueue Element(queue=w444, element=w442, error in (no error)=w445) -> (error out=w440:errorcluster)  [unwired: 1 in, 2 out]
      }
      frame "Quit" {
        n154 = Generate User Event(user event=w459, event data cluster=TRUE ("event data"), error in=w458) -> (error out=w457:errorcluster)  [unwired: 1 in, 1 out]
      }
      frame "gRPC_Update-PumpCtrl" {
        n155 = Unbundle By Name(w465) -> ("Node Info.Connected?"=w464:bool)
        n156 = case shown="True" w464 {
          tunnel: w472 -> [w474 w485]
          tunnel: [w473 w484] -> w471
          tunnel: [w474 w483] -> w470
          tunnel: w469 -> [_ w482]
          tunnel: w468 -> [w473 w481]
          tunnel: w465 -> [w475 w478]
          tunnel: [w475 w476] -> w467
          frame False {
          }
          frame True {
            n157 = Variant To Data(error in=w481, type=T4 {"Pump Enable"=FALSE, "Demand"=0.0, "Sump Pump Enable"=FALSE} ("Pump Control"), Variant=w482) -> (data=w477:T4, error out=w480:errorcluster)
            n158 = Unbundle(w477) -> ("Pump Enable"=w487:bool, "Demand"=w486:dbl, "Sump Pump Enable"=w490:bool)
            n159 = Bundle(cluster=T19 {"pumpEnable"=FALSE, "pumpDemand"=0.0, "sumppumpEnable"=FALSE} ("System Control Request"), "pumpEnable"=w487, "pumpDemand"=w486, "sumppumpEnable"=w490) -> (w488:T19)
            n160 = Bundle By Name(cluster=w478, "Pump Control"=w477) -> (w476:T12)
            n161 = call "PumpController SetSystemControl.vi"("error in"=w480, "Request Data"=w488, "gRPC ID"=w485) -> ("error out"=w484:errorcluster, "gRPC ID out"=w483:T6)  [unwired: 6 in, 1 out]
          }
        }
      }
      frame "gRPC_Update-ValveCtrl" {
        n162 = Unbundle By Name(w491) -> ("Node Info.Connected?"=w492:bool)
        n163 = case shown="True" w492 {
          tunnel: w499 -> [_ w524]
          tunnel: w498 -> [w500 w523]
          tunnel: w491 -> [w502 w521]
          tunnel: [w502 w504] -> w497
          tunnel: w496 -> [w501 w514]
          tunnel: [w500 w508] -> w495
          tunnel: [w501 w507] -> w494
          frame False {
          }
          frame True {
            n164 = Variant To Data(error in=w523, type=T5 {"Tank Fill"=FALSE, "Tank Outlet"=FALSE, "Tank Drain"=FALSE, "DUT Inlet"=FALSE, "DUT Outlet"=FALSE, "Sump Drain"=FALSE, "Tank Fill Open"=FALSE, "Tank Fill Closed"=FALSE, "Tank Outlet Open"=FALSE, "Tank Outlet Closed"=FALSE, "Tank Drain Open"=FALSE, "Tank Drain Closed"=FALSE, "DUT Inlet Open"=FALSE, "DUT Inlet Closed"=FALSE, "DUT Outlet Open"=FALSE, "DUT Outlet Closed"=FALSE, "Sump Drain Open"=FALSE, "Sump Drain Closed"=FALSE} ("Control Valves"), Variant=w524) -> (data=w520:T5, error out=w513:errorcluster)
            n165 = Unbundle By Name(w520) -> ("Tank Fill"=w525:bool, "Tank Outlet"=w518:bool, "Tank Drain"=w526:bool, "DUT Inlet"=w517:bool, "DUT Outlet"=w516:bool, "Sump Drain"=w515:bool)
            n166 = Bundle By Name(cluster=w521, "Control Valves"=w520) -> (w504:T12)
            n167 = Bundle By Name(cluster=T16 {"tankFillIV"=FALSE, "tankOutIV"=FALSE, "tankDrainIV"=FALSE, "dutInIV"=FALSE, "dutOutIV"=FALSE, "sumpDrainIV"=FALSE} ("Valve Control Request"), "tankFillIV"=w525, "tankOutIV"=w518, "tankDrainIV"=w526, "dutInIV"=w517, "dutOutIV"=w516, "sumpDrainIV"=w515) -> (w512:T16)
            n168 = call "PumpController SetValveStatus.vi"("error in"=w513, "Request Data"=w512, "gRPC ID"=w514) -> ("error out"=w510:errorcluster, "gRPC ID out"=w509:T6)  [unwired: 6 in, 1 out]
            n169 = Unbundle By Name(w504) -> ("Control Valves"=w503:T5)
            n170 = call "PumpController GetValveStatus.vi"("error in"=w510, "Request Data"=T15 {"request"=FALSE}, "gRPC ID"=w509) -> ("error out"=w508:errorcluster, "Response Data"=w511:T16, "gRPC ID out"=w507:T6)  [unwired: 6 in]
            n171 = call "Handle Valve Status.vi"("Response Data"=w511, "Control Valves in"=w503) -> ("Control Valves out"=w505:T5)  [unwired: 9 in]
            n172 = property on="Control Valves" class="Clust (strict)"("Value"=w505) -> ()  [unwired: 2 in, 2 out]
          }
        }
      }
      frame "gRPC_ReadAll" {
        n173 = Unbundle By Name(w528) -> ("Node Info.Connected?"=w527:bool)
        n174 = case shown="False" w527 {
          tunnel: w534 -> [w537 w556]
          tunnel: [w537 w540] -> w533
          tunnel: [w536 w541] -> w532
          tunnel: w531 -> [w536 w555]
          tunnel: w528 -> [w535 w549]
          tunnel: [w535 w547] -> w530
          frame False {
          }
          frame True {
            n175 = call "PumpController GetSystemInfo.vi"("error in"=w556, "Request Data"=T13 {"request"=FALSE}, "gRPC ID"=w555) -> ("error out"=w538:errorcluster, "Response Data"=w554:T14, "gRPC ID out"=w539:T6)  [unwired: 6 in]
            n176 = Unbundle(w554) -> ("nodeID"=w553:i32, "statusMsg"=w552:string)  [unwired: 1 out]
            n177 = Unbundle By Name(w549) -> ("Node Info"=w548:T1)  [unwired: 1 out]
            n178 = Number To Decimal String(number=w553) -> (decimal integer string=w551:string)  [unwired: 1 in]
            n179 = Empty String/Path?(string/path=w551) -> (empty?=w543:bool)
            n180 = Not(x=w543) -> (.not. x?=w542:bool)
            n181 = Bundle By Name(cluster=w548, "Connected?"=w542, "Status"=w552) -> (w550:T1)
            n182 = call "PumpController GetSensorReading.vi"("error in"=w538, "Request Data"=T17 {"request"=FALSE}, "gRPC ID"=w539) -> ("error out"=w540:errorcluster, "Response Data"=w546:T20, "gRPC ID out"=w541:T6)  [unwired: 6 in]
            n183 = Bundle By Name(cluster=w549, "Node Info"=w550, "Sensors"=w546) -> (w547:T12)
          }
        }
      }
      frame "gRPC_Stream-Start" {
        n184 = Enqueue Element(queue=w562, element=T9 {"Enum"=enum."gRPC_StartStream", variant}, error in (no error)=w564) -> (error out=w563:errorcluster)  [unwired: 1 in, 2 out]
        n185 = Bundle By Name(cluster=w560, "Streaming"=TRUE) -> (w559:T12)
      }
      frame "gRPC_Stream-Stop" {
        n186 = Enqueue Element(queue=w571, element=T9 {"Enum"=enum."gRPC_StopStream", variant}, error in (no error)=w573) -> (error out=w572:errorcluster)  [unwired: 1 in, 2 out]
        n187 = Bundle By Name(cluster=w569, "Streaming"=FALSE) -> (w568:T12)
      }
    }
    "gRPC ID Out" <- w338
    n188 = Unbundle By Name(w346) -> ("Node Info"=w345:T1, "Sensors"=w344:T2, "Node Info.Connected?"=w335:bool, "Streaming"=w333:bool)  [unwired: 2 out]
    n189 = Not(x=w333) -> (.not. x?=w334:bool)
    n190 = And(x=w335, y=w334) -> (x .and. y?=w332:bool)
    n191 = case shown="False" w332 {
      tunnel: w342 -> [_ w358]
      tunnel: [w355 w357] -> w341
      tunnel: w339 -> [w355 w356]
      frame False {
      }
      frame True {
        n192 = Bundle(cluster=T11 {enum."Initialise", variant}, States."gRPC_ReadAll") -> (w360:T11)  [unwired: 1 in]
        n193 = Enqueue Element(queue=w358, element=w360, error in (no error)=w356) -> (error out=w357:errorcluster)  [unwired: 1 in, 2 out]
      }
    }
    n194 = property on="Node Info" class="Clust (strict)"(error in=w341, "Value"=w345) -> ()  [unwired: 1 in, 2 out]
    n195 = property on="Sensors" class="Clust (strict)"(error in=w341, "Value"=w344) -> ()  [unwired: 1 in, 2 out]
    n196 = flat-sequence {
      tunnel: [w362] -> w340
      tunnel: w341 -> [w362]
      frame #0 {
        n197 = Wait (ms)(milliseconds to wait=u32 100) -> ()  [unwired: 1 out]
      }
    }
  }
  n198 = while {
    tunnel: w25 -> [w577]
    tunnel: w8 -> [w582]
    tunnel: [w579] -> w20
    tunnel: w21 -> [w576]
    tunnel: w1 -> [w575]
    stop <- w581 stop-if-true
    # "Producer Loop"
    n199 = event shown="[9] <Stop>: User Event" {
      selector: w576 -> [_ _ _ _ _ _ _ _ _ w654]
      dyn-events: _ -> [_ _ _ _ _ _ _ _ _ _]
      timeout: _ -> [_ _ _ _ _ _ _ _ _ _]
      tunnel: w577 -> [_ w585 w592 w598 w605 w615 w620 w628 w643 w652]
      tunnel: w582 -> [w583 w586 w593 w599 w606 w616 w621 w629 w641 w651]
      tunnel: [w583 w587 w594 w600 w607 w617 w622 w630 w637 w653] -> w579
      tunnel: [_ _ _ _ _ _ _ _ _ TRUE ("Stop")] -> w580
      tunnel: w575 -> [_ _ _ _ _ _ _ _ w642 w647]
      event Timeout {
        n200 = event-data() -> ()  [unwired: 1 in, 3 out]
      }
      event Value Change {
        n201 = event-data() -> ()  [unwired: 1 in, 6 out]
        n202 = Bundle(cluster=T11 {enum."Initialise", variant}, States."gRPC_Update-ValveCtrl", "Control Valves") -> (w588:T11)
        n203 = Enqueue Element(queue=w585, element=w588, error in (no error)=w586) -> (error out=w587:errorcluster)  [unwired: 1 in, 2 out]
      }
      event Value Change {
        n204 = event-data() -> ()  [unwired: 1 in, 6 out]
        n205 = Bundle(cluster=T11 {enum."Initialise", variant}, States."gRPC_Update-PumpCtrl", "Pump Control") -> (w595:T11)
        n206 = Enqueue Element(queue=w592, element=w595, error in (no error)=w593) -> (error out=w594:errorcluster)  [unwired: 1 in, 2 out]
      }
      event "gRPC Connect": Value Change {
        n207 = event-data() -> ()  [unwired: 1 in, 6 out]
        n208 = Bundle(cluster=T11 {enum."Initialise", variant}, States."gRPC_Connect") -> (w601:T11)  [unwired: 1 in]
        n209 = Enqueue Element(queue=w598, element=w601, error in (no error)=w599) -> (error out=w600:errorcluster)  [unwired: 1 in, 2 out]
      }
      event "Server Address": Value Change {
        n210 = event-data() -> ()  [unwired: 1 in, 6 out]
        n211 = Bundle(cluster=T11 {enum."Initialise", variant}, States."Update Settings", "Server Address") -> (w608:T11)
        n212 = Enqueue Element(queue=w605, element=w608, error in (no error)=w606) -> (error out=w607:errorcluster)  [unwired: 1 in, 2 out]
      }
      event "Stream Enable": Value Change {
        n213 = event-data() -> ()  [unwired: 1 in, 6 out]
        n214 = Select(t=States."gRPC_Stream-Start", s="Stream Enable", f=States."gRPC_Stream-Stop") -> (s? t:f=w611:T10)
        n215 = Bundle(cluster=T11 {enum."Initialise", variant}, w611) -> (w618:T11)  [unwired: 1 in]
        n216 = Enqueue Element(queue=w615, element=w618, error in (no error)=w616) -> (error out=w617:errorcluster)  [unwired: 1 in, 2 out]
      }
      event "gRPC Disconnect": Value Change {
        n217 = event-data() -> ()  [unwired: 1 in, 6 out]
        n218 = Bundle(cluster=T11 {enum."Initialise", variant}, States."gRPC_Disconnect") -> (w623:T11)  [unwired: 1 in]
        n219 = Enqueue Element(queue=w620, element=w623, error in (no error)=w621) -> (error out=w622:errorcluster)  [unwired: 1 in, 2 out]
      }
      event "Apply Preset": Value Change {
        n220 = event-data() -> ()  [unwired: 1 in, 6 out]
        n221 = case shown="\"Home WiFi\"" "Address Presets" {
          tunnel: ["" "192.168.0.141:50051" "10.42.0.1:50051"] -> w626
          frame Default {
          }
          frame "Home WiFi" {
          }
          frame "RasPi WiFi" {
          }
        }
        n222 = Bundle(cluster=T11 {enum."Initialise", variant}, States."Update Settings", w626) -> (w631:T11)
        n223 = Enqueue Element(queue=w628, element=w631, error in (no error)=w629) -> (error out=w630:errorcluster)  [unwired: 1 in, 2 out]
      }
      event "Stop": Value Change {
        n224 = event-data() -> ()  [unwired: 1 in, 6 out]
        n225 = Enqueue Element(queue=w642, element=T9 {"Enum"=enum."Stop", variant}, error in (no error)=w641) -> (error out=w638:errorcluster)  [unwired: 1 in, 2 out]
        n226 = Bundle(cluster=T11 {enum."Initialise", variant}, States."Stop") -> (w644:T11)  [unwired: 1 in]
        n227 = Enqueue Element(queue=w643, element=w644, error in (no error)=w641) -> (error out=w639:errorcluster)  [unwired: 1 in, 2 out]
        n228 = Merge Errors(w638, w639) -> (w637:errorcluster)
      }
      event User Event {
        n229 = event-data() -> ()  [unwired: 1 in, 4 out]
        n230 = Release Queue(queue=w647, error in (no error)=w651) -> (error out=w650:errorcluster)  [unwired: 1 in, 2 out]
        n231 = Release Queue(queue=w652, error in (no error)=w651) -> (error out=w649:errorcluster)  [unwired: 1 in, 2 out]
        n232 = Merge Errors(w650, w649) -> (w648:errorcluster)
        n233 = Unregister For Events(event registration refnum=w654, error in=w648) -> (error out=w653:errorcluster)
      }
    }
    n234 = Unbundle By Name(w579) -> ("status"=w578:bool)
    n235 = Or(x=w578, y=w580) -> (x .or. y?=w581:bool)
  }
  n236 = Destroy User Event(user event=w16, error in=w20) -> (error out=w19:errorcluster)
  n237 = Merge Errors(w32, w19, w6) -> (w31:errorcluster)
  n238 = call <vilib>:"Simple Error Handler.vi"("error in (no error)"=w31) -> ("error out"=w30:errorcluster)  [unwired: 4 in, 4 out]
  n239 = call <vilib>:"Clear Errors.vi"("error in (no error)"=w30) -> ("error out"=→"Error":errorcluster)  [unwired: 5 in, 1 out]
